vi "Pinball Up.vi"() -> ()   [LabVIEW 2019]
uses:
  <vilib>/Rock Robotics/WPI/Framework/Command Status Info.ctl
  <vilib>/Rock Robotics/WPI/Framework/Completion Status.ctl
  <vilib>/Rock Robotics/WPI/Framework/Completion Notifier.ctl
  Implementation/Ball Intake Setpoints.ctl
  Implementation/Ball Intake Operations.ctl
panel:
  in  "Description":string
  out "Command Info Out":T1
  in  "Command Info In":T1
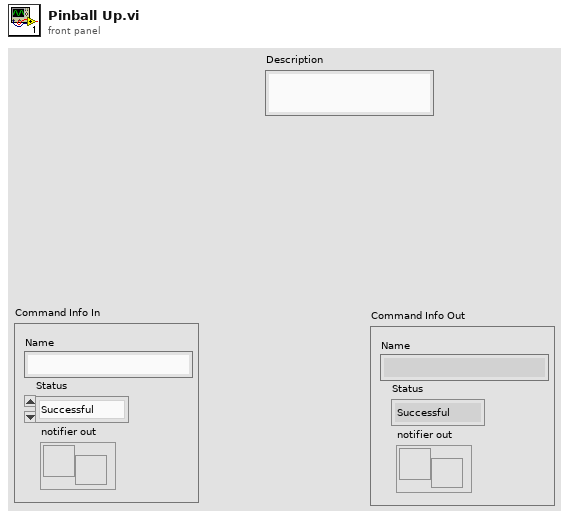
[diagram p1: front panel]
types:
  T1 = typedef "Command Status Info.ctl" = cluster{"Name":string, "Status":T2, "notifier out":T3}
  T2 = typedef "Completion Status.ctl" = enum16{"Successful", "Aborted", "Incomplete"}
  T3 = typedef "Completion Notifier.ctl" = refnum<notifier>
  T4 = typedef "Ball Intake Setpoints.ctl" = cluster{"Operation":T5, "Setpoint":dbl, "Duration":dbl, "Setpoint 2":dbl, "Open/Close":bool}
  T5 = typedef "Ball Intake Operations.ctl" = enum16{"Reserve", "Read Current", "Ball intake operation", "Pinball Up", "Pinball Down", "Immediate"}
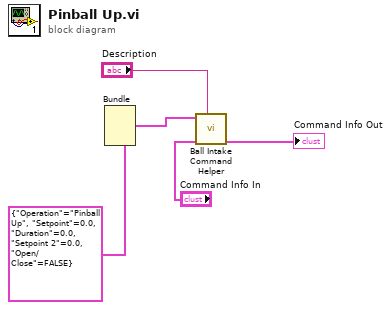
[diagram p0: block diagram]
diagram:
  n1 = Bundle(cluster=T4 {"Operation"=enum."Pinball Up", "Setpoint"=0.0, "Duration"=0.0, "Setpoint 2"=0.0, "Open/Close"=FALSE} ("SubSystem Data")) -> (w1:T4)  [unwired: 5 in]
  n2 = call "Ball Intake Command Helper.vi"("Description"="Description", "Command Info In"="Command Info In", "SubSystem Data"=w1) -> ("Command Info Out"=→"Command Info Out":T1)  [unwired: 6 in, 2 out]
